vi "User Continue.vi"(10 "Enable":bool, 11 "Msg input":string) -> (3 "Continue":bool)   [LabVIEW 2015]
panel:
  in  "Continue":bool
  in  "Ignore":bool
  out "Msg":string
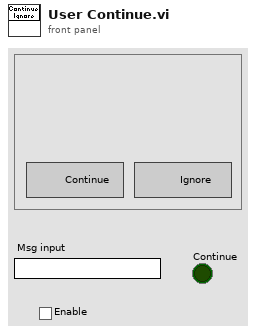
[diagram p1: front panel]
types:
  T1 = enum32{"Invalid", "Standard", "Closed", "Hidden", "Minimized", "Maximized"}
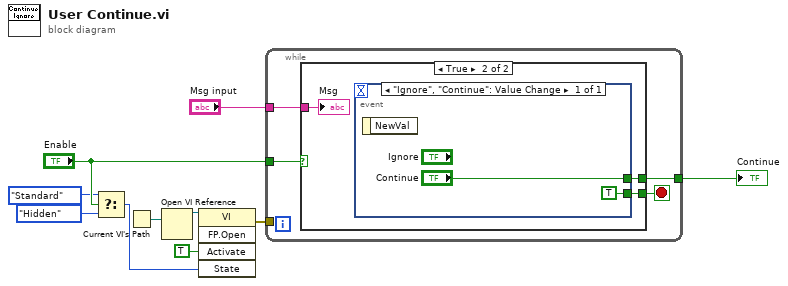
[diagram p0: block diagram]
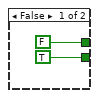
[diagram p2: hidden frame]
diagram:
  n1 = Select(t=T1."Standard" ("State"), s="Enable", f=T1."Hidden" ("State")) -> (s? t:f=w1:T1)
  n2 = Current VI's Path() -> (path=w8:path)
  n3 = Open VI Reference(vi path=w8) -> (vi reference=w7:refnum<vi>)  [unwired: 5 in, 1 out]
  n4 = invoke class="VI" method="FP.Open"(reference=w7, "Activate"=TRUE ("Activate?"), "State"=w1) -> (error out=w6:errorcluster)  [unwired: 2 in, 4 out]
  n5 = while {
    tunnel: [w14] -> w10
    tunnel: "Msg input" -> [w12]
    tunnel: "Enable" -> [w11]
    tunnel: w6 -> [_]
    stop <- w13 stop-if-true
    n6 = case shown="True" w11 {
      tunnel: [FALSE ("Continue") w19] -> w14
      tunnel: [TRUE w18] -> w13
      tunnel: w12 -> [_ w17]
      frame False {
      }
      frame True {
        n7 = event shown="[0] \"Ignore\", \"Continue\": Value Change" {
          selector: _ -> [_]
          dyn-events: _ -> [_]
          timeout: _ -> [_]
          tunnel: ["Continue"] -> w19
          tunnel: [TRUE] -> w18
          event "Ignore", "Continue": Value Change {
            n8 = event-data() -> ()  [unwired: 1 in, 1 out]
          }
        }
        "Msg" <- w17
      }
    }
  }
  "Continue" <- w10
